vi "Initialize.vi"(8 "error in (no error)":errorcluster, 11 "Simulated Device in":refnum<class "Simulated Device.lvclass">) -> (0 "error out":errorcluster, 2 "Connected?":bool, 3 "Simulated Device out":refnum<class "Simulated Device.lvclass">)   [LabVIEW 2020, in "Simulated Device.lvclass"]
doc: "Initialize a device."
uses:
  Simulated Device.lvclass
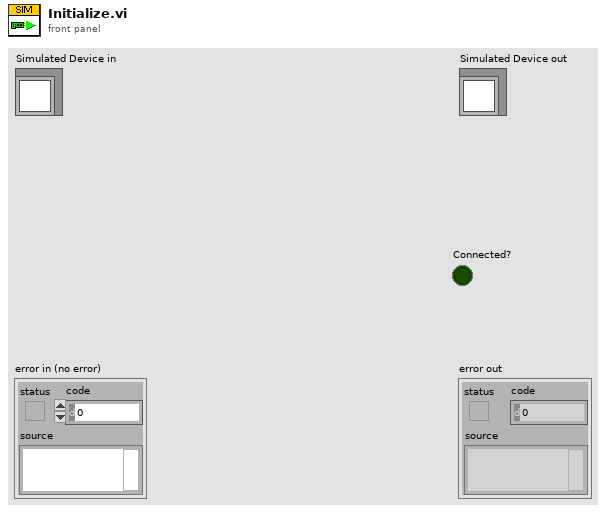
[diagram p1: front panel]
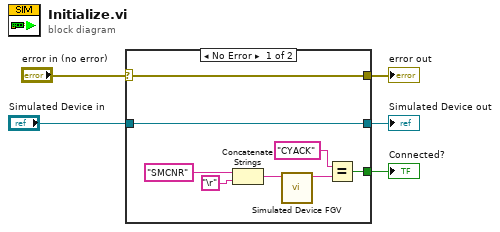
[diagram p0: block diagram]
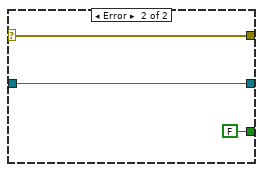
[diagram p2: hidden frame]
diagram:
  n1 = case shown="No Error" "error in (no error)" {
    selector: "error in (no error)" -> [w8 w15]
    tunnel: [w9 w16] -> w4
    tunnel: "Simulated Device in" -> [w9 w16]
    tunnel: [w8 w15] -> w2
    tunnel: [w12 FALSE] -> w1
    frame No Error {
      n2 = Concatenate Strings("SMCNR" ("write buffer"), "\r") -> (w7:string)
      n3 = call "Simulated Device FGV.vi"("Request"=w7) -> ("Response"=w6:string)  [unwired: 10 in]
      n4 = Equal?(x="CYACK", y=w6) -> (x = y?=w12:bool)
    }
    frame Error {
    }
  }
  "error out" <- w2
  "Simulated Device out" <- w4
  "Connected?" <- w1
